vi "LS4 SetControlParsSD.vi"() -> (0 "Command executed":bool)   [LabVIEW 2015]
doc: "Sends the LStep parameters. These can be loaded by LS4 LoadConfig.vi or edited by LS4 AxisParsDlg.vi / LS4 ControllerParsDlg.vi."
uses:
  DLL/LStep4.dll
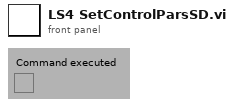
[diagram p1: front panel]
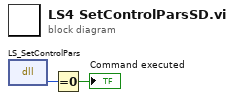
[diagram p0: block diagram]
diagram:
  n1 = dll-call lib="G:/SD/TRANCON-2015/DLL/LStep4.dll" fn="LS_SetControlPars"() -> ("type de retour"=w2:i32)  [unwired: 3 in, 2 out]
  n2 = Equal To 0?(x=w2) -> (x = 0?=→"Command executed":bool)
